vi "Prune.vi"(11 "Secret Number":u64) -> (3 "New Secret Number":u64)   [LabVIEW 2024]
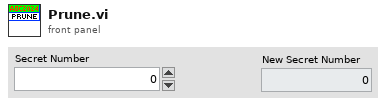
[diagram p1: front panel]
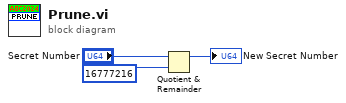
[diagram p0: block diagram]
diagram:
  n1 = Quotient & Remainder(x="Secret Number", y=u64 16777216) -> (x-y*floor(x/y)=→"New Secret Number":u64)  [unwired: 1 out]
